vi "TemperatureControl.vi"(8 "error in (no error)":errorcluster, 11 "VISA resource name":refnum<visa-resource-name>="itcetherT") -> (0 "error out":errorcluster)   [LabVIEW 2017]
uses:
  controls/iTCsetCtrl.ctl
  controls/iTCreadCtrl.ctl
  <vilib>/Instr/_visa.llb/VISA Open Access Mode.ctl
panel:
  out "Waveform Chart":T1(graph)
  out "Signals":string[](array[string])=["PT1 (K)", "PT2 (K)", "Sample_T (K)", "VTI_T (K)", "Needle Valve (%)", "VTI Heater P", "Sample Heater P ", "VTI Pressure (mBar)"]
  out "Temperature Readings":dbl[](array[numeric])
  in  "Setpoint":dbl
  in  "iTCreadCtrl":T2
  in  "iTCSetCtrl":T3
  in  "Set":bool
  in  "Refresh Time (ms)":i32=100
  in  "Quit":bool
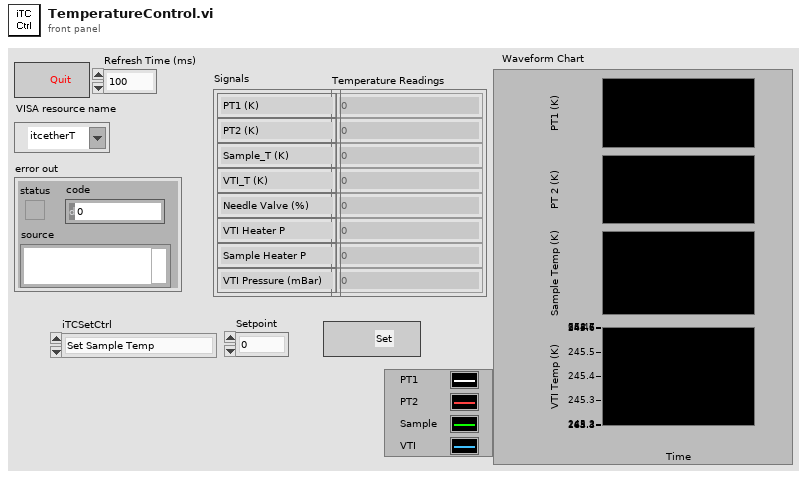
[diagram p1: front panel]
types:
  T1 = cluster{"number":dbl, "number":dbl, "number":dbl, "number":dbl}
  T2 = typedef "iTCreadCtrl.ctl" = enum16{"PT1 Temp", "PT2 Temp", "Sample Temp", "VTI Temp", "Needle Valve", "VTI Heater Power", "Sample Heater Power", "VTI Pressure"}
  T3 = typedef "iTCsetCtrl.ctl" = enum16{"Set Sample Temp", "Set VTI Temp", "Set Needle Valve", "Set VTI Heater Power", "Set Sample Heater Power", "Set VTI Pressure"}
  T4 = typedef "VISA Open Access Mode.ctl" = u32
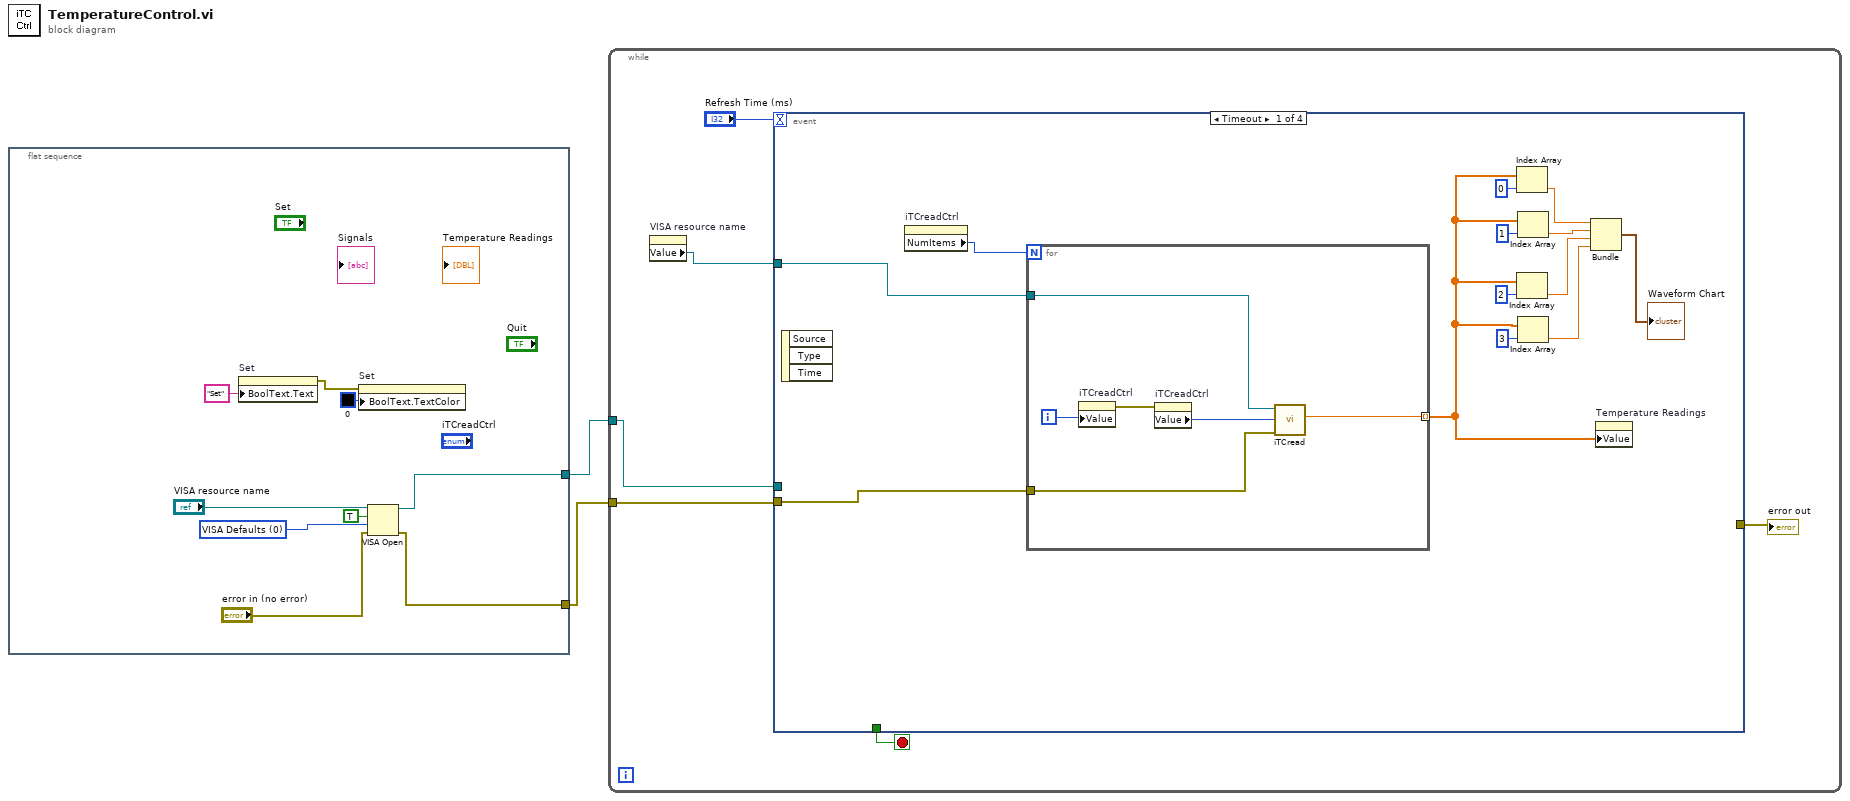
[diagram p0: block diagram]
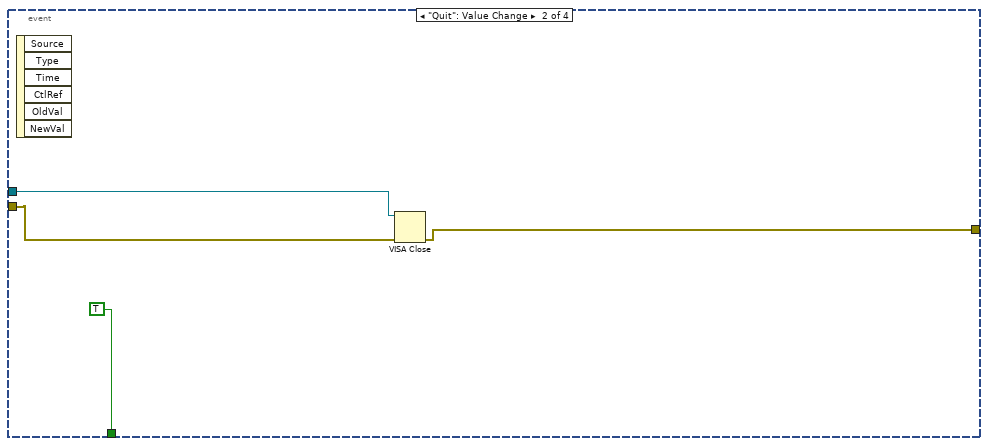
[diagram p2: hidden frame]
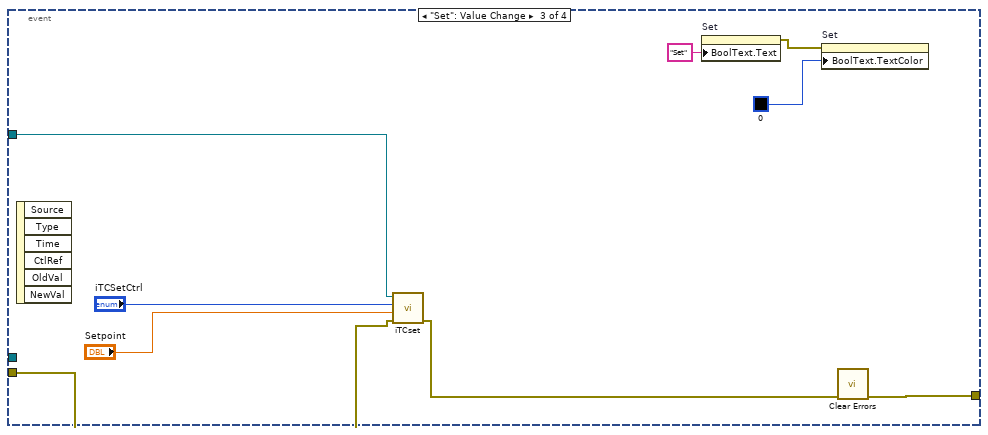
[diagram p3: hidden frame]
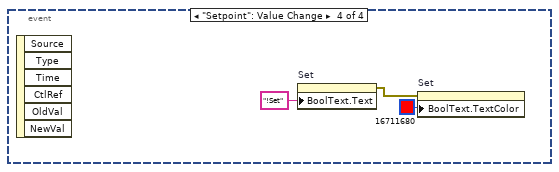
[diagram p4: hidden frame]
diagram:
  n1 = flat-sequence {
    tunnel: [w7] -> w2
    tunnel: [w4] -> w1
    frame #0 {
      w3 = T4 0 items=["VISA Defaults"=0, "Exclusive Lock"=1, "Load Configured Settings"=4] ("Access Mode")
      n2 = property on="Set" class="Bool (strict)"("BoolText.Text"="Set" ("Boolean Text.Text")) -> (error out=w11:errorcluster)  [unwired: 2 in, 1 out]
      n3 = property on="Set" class="Bool (strict)"(error in=w11, "BoolText.TextColor"=u32 0 ("Boolean Text.Colors:BG Color")) -> ()  [unwired: 1 in, 2 out]
      n4 = VISA Open(duplicate session (F)=TRUE, access mode=w3, error in (no error)="error in (no error)", VISA resource name="VISA resource name") -> (VISA resource name=w4:refnum<visa-resource-name>, error out=w7:errorcluster)  [unwired: 1 in]
    }
  }
  n5 = while {
    tunnel: w2 -> [w16]
    tunnel: w1 -> [w13]
    stop <- w15 stop-if-true
    n6 = property on="VISA resource name" class="VISAName"() -> ("Value"=w12:refnum<visa-resource-name>)  [unwired: 2 in, 2 out]
    n7 = event shown="[0] Timeout" {
      selector: _ -> [_ _ _ _]
      dyn-events: _ -> [_ _ _ _]
      timeout: "Refresh Time (ms)" -> [_ _ _ _]
      tunnel: w16 -> [w30 w39 w45 _]
      tunnel: [_ w38 w49 _] -> w14
      tunnel: w12 -> [w29 _ w48 _]
      tunnel: [_ TRUE _ _] -> w15
      tunnel: w13 -> [_ w37 _ _]
      event Timeout {
        n8 = event-data() -> ()  [unwired: 1 in, 3 out]
        n9 = property on="iTCreadCtrl" class="Enum (strict)"() -> ("NumItems"=w28:u32)  [unwired: 2 in, 2 out]
        n10 = for {
          N: w28 -> [_]
          tunnel: w30 -> [w36]
          tunnel: w29 -> [w35]
          tunnel: [w31] -> w23 mode=indexing
          i -> [w34]
          n11 = property on="iTCreadCtrl" class="Enum (strict)"("Value"=w34) -> (error out=w33:errorcluster)  [unwired: 2 in, 1 out]
          n12 = property on="iTCreadCtrl" class="Enum (strict)"(error in=w33) -> ("Value"=w32:T2)  [unwired: 1 in, 2 out]
          n13 = call "iTCread.vi"("VISA resource name"=w35, "iTCreadCtrl"=w32, "error in (no error)"=w36) -> ("number"=w31:dbl)  [unwired: 4 in, 3 out]
        }
        n14 = Index Array(array=w23, index=0) -> (element=w22:dbl)
        n15 = Index Array(array=w23, index=2) -> (element=w20:dbl)
        n16 = Index Array(array=w23, index=1) -> (element=w21:dbl)
        n17 = Index Array(array=w23, index=3) -> (element=w19:dbl)
        n18 = Bundle("number"=w22, "number"=w21, "number"=w20, "number"=w19) -> (→"Waveform Chart":T1)  [unwired: 1 in]
        n19 = property on="Temperature Readings" class="Arr (strict)"("Value"=w23) -> ()  [unwired: 2 in, 2 out]
      }
      event "Quit": Value Change {
        n20 = event-data() -> ()  [unwired: 1 in, 6 out]
        n21 = VISA Close(VISA resource name=w37, error in (no error)=w39) -> (error out=w38:errorcluster)
      }
      event "Set": Value Change {
        n22 = event-data() -> ()  [unwired: 1 in, 6 out]
        n23 = call "iTCset.vi"("error in (no error)"=w45, "Set Point"="Setpoint", "iTCSetCtrl"="iTCSetCtrl", "VISA resource name"=w48) -> ("error out"=w44:errorcluster)  [unwired: 4 in, 3 out]
        n24 = property on="Set" class="Bool (strict)"("BoolText.Text"="Set" ("Boolean Text.Text")) -> (error out=w41:errorcluster)  [unwired: 2 in, 1 out]
        n25 = property on="Set" class="Bool (strict)"(error in=w41, "BoolText.TextColor"=u32 0 ("Boolean Text.Colors:BG Color")) -> ()  [unwired: 1 in, 2 out]
        n26 = call <vilib>:"Clear Errors.vi"("error in (no error)"=w44) -> ("error out"=w49:errorcluster)  [unwired: 5 in, 1 out]
      }
      event "Setpoint": Value Change {
        n27 = event-data() -> ()  [unwired: 1 in, 6 out]
        n28 = property on="Set" class="Bool (strict)"("BoolText.Text"="!Set" ("Boolean Text.Text")) -> (error out=w51:errorcluster)  [unwired: 2 in, 1 out]
        n29 = property on="Set" class="Bool (strict)"(error in=w51, "BoolText.TextColor"=u32 16711680 ("Boolean Text.Colors:BG Color")) -> ()  [unwired: 1 in, 2 out]
      }
    }
    "error out" <- w14
  }
